vi "test_Create Data Channel_single channel type cast .vi"(8 "error in (no error)":errorcluster, 11 "TestCase in":refnum<class "Instrument Addon Scripting API Channels Unit Tests.lvclass">) -> (0 "error out":errorcluster, 3 "TestCase out":refnum<class "Instrument Addon Scripting API Channels Unit Tests.lvclass">)   [LabVIEW 2018, in "Instrument Addon Scripting API Channels Unit Tests.lvclass"]
uses:
  Instrument Addon Scripting API Channels Unit Tests.lvclass
  APIs/Scripting API/TypeDefs/Single Channel Type Cast Settings.ctl
  Addon/Addon Shared/Types/Type Cast Type.ctl
  Addon/Addon Shared/Types/Endian.ctl
  Addon/Addon Shared/Types/Protocol Data Type.ctl
  Addon/Addon Shared/Types/Data Channel Type.ctl
  Instrument Addon Scripting API Channels Unit Tests.lvclass/Instrument Addon Scripting API Channels Unit Tests.ctl
  Addon/Addon Shared/SubVIs/Constants.vi
  <vilib>/NI/NI VeriStand Advanced SysDef API/_SubVIs/SysDef.Search.GUID.vi
  <vilib>/NI/NI VeriStand Advanced SysDef API/_SubVIs/SysDef.Search.GUIDs.vi
  APIs/Scripting API/Channels/Create Data Channel - Single Channel - Type Cast.vi
  <vilib>/NI Veristand/Custom Device API/Get Item Property (U16).vi
  <vilib>/addons/_JKI Toolkits/VI Tester/TestCase.llb/TestCase.lvclass
  Instrument Addon Scripting API Test Assets/Instrument Addon Scripting API Test Assets.lvclass
  <vilib>/NI/NI VeriStand Advanced SysDef API/SysDef API/Advanced System Definition.lvlib
  Addon/Addon Shared/Instrument Addon Shared.lvlib
  <vilib>/NI Veristand/Custom Device API/Custom Device API.lvlib
  APIs/Scripting API/Instrument Addon Scripting API.lvlib
  C:/Program Files (x86)/National Instruments/LabVIEW 2018/vi.lib/addons/_JKI Toolkits/VI Tester/TestCase.llb/TestCase.lvclass
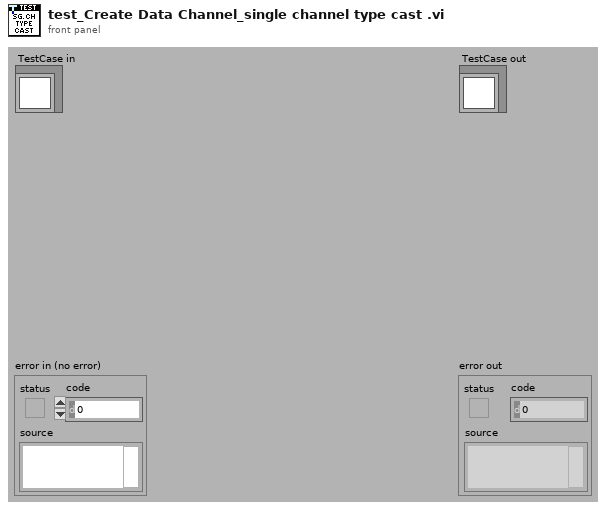
[diagram p1: front panel]
types:
  T1 = typedef "Instrument Addon Scripting API.lvlib/Single Channel Type Cast Settings.ctl" = cluster{"Type":T2, "Endian":T3, "Default Value":dbl, "Units":string}
  T2 = typedef "Instrument Addon Shared.lvlib/Type Cast Type.ctl" = enum16{"DBL", "SGL", "U64", "U32", "U16", "U8", "I64", "I32", "I16", "I8"}
  T3 = typedef "Instrument Addon Shared.lvlib/Endian.ctl" = enum16{"Native", "Little", "Big"}
  T4 = typedef "Instrument Addon Shared.lvlib/Data Channel Type.ctl" = enum16{"Format", "Comparison", "Type Cast", "Enumerated List"}
  T5 = typedef "Instrument Addon Shared.lvlib/Protocol Data Type.ctl" = enum16{"Single Channel", "Array"}
  T6 = typedef "Custom Device API.lvlib/Custom Device Item Ref.ctl" = u64
  T7 = typedef "Custom Device API.lvlib/Custom Device Channel.ctl" = cluster{"Type":T8, "Units":string, "Default Value":dbl, "Faultable":bool, "Scalable":bool}
  T8 = typedef "Custom Device API.lvlib/Custom Device Channel Type.ctl" = enum16{"Input", "Output"}
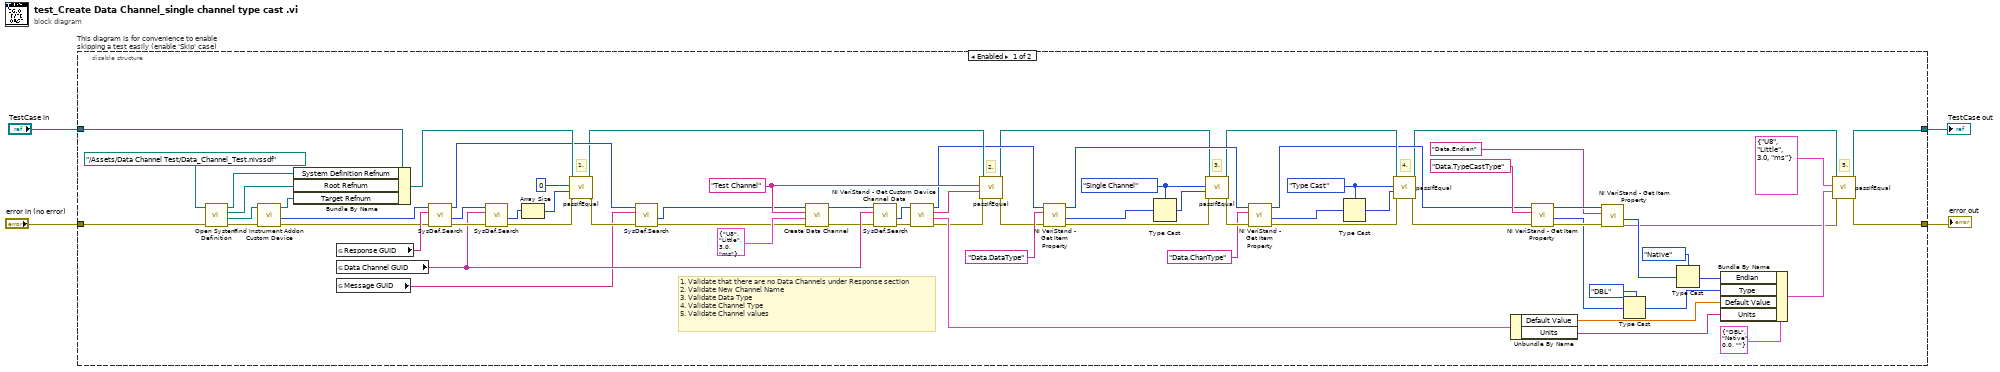
[diagram p0: block diagram]
diagram:
  n1 = disable-structure "This diagram is for convenience to enable skipping a test easily (enable 'Skip' case)" shown="Enabled" {
    disable-tunnel: "TestCase in" -> [w37 w79]
    disable-tunnel: [w75 w77] -> w1
    disable-tunnel: [w74 w78] -> w3
    disable-tunnel: "error in (no error)" -> [w70 w76]
    frame Enabled {
      w15 = Data_Channel_Type."Type Cast" ("Channel Type")
      w20 = Protocol_Data_Type."Single Channel" ("Data Type")
      w54 = "Test Channel" ("Name")
      # "2."
      # "4."
      # "3."
      # "5."
      # "1. Validate that there are no Data Channels under Response section\n2. Validate New Channel Name\n3. Validate Data Type\n4. Validate Channel Type\n5. Validate Channel values"
      # "1."
      n2 = call "Open System Definition.vi"("error in (no error)"=w70, "System Definition File"=path "../Assets/Data Channel Test/Data_Channel_Test.nivssdf") -> ("error out"=w73:errorcluster, "Target Refnum"=w72:refnum<k24>, "Root Refnum"=w34:refnum<k24>, "System Definition Refnum"=w36:refnum<k24>)  [unwired: 6 in]
      n3 = call "Find Instrument Addon Custom Device.vi"("error in"=w73, "target in"=w72) -> ("error out"=w38:errorcluster, "NodeID"=w30:u64, "target out"=w33:refnum<k24>)  [unwired: 7 in]
      n4 = Bundle By Name(cluster=w37, "System Definition Refnum"=w36, "Root Refnum"=w34, "Target Refnum"=w33) -> (w35:refnum<class "Instrument Addon Scripting API Channels Unit Tests.lvclass">)
      n5 = global read "Constants.vi" "Response GUID"() -> (w69:string)
      n6 = global read "Constants.vi" "Data Channel GUID"() -> (w66:string)
      n7 = global read "Constants.vi" "Message GUID"() -> (w31:string)
      n8 = call-poly <vilib>:"SysDef.Search.vi"("error in (no error)"=w38, "GUID"=w69, "nodeID"=w30) -> ("error out"=w67:errorcluster, "Value out"=w68:u64, "nodeID out"=w27:u64)  [unwired: 5 in, 1 out]
      n9 = call-poly <vilib>:"SysDef.Search.vi"("error in (no error)"=w67, "GUID"=w66, "nodeID"=w68) -> ("error out"=w58:errorcluster, "Values Out"=w57:u64[])  [unwired: 5 in, 2 out]
      n10 = Array Size(array=w57) -> (size(s)=w56:i32)
      n11 = call-dynamic "passIfEqual.vi"("error in (no error)"=w58, "y"=w56, "x"=0 ("size(s)"), "TestCase in"=w35) -> ("error out"=w32:errorcluster, "TestCase out"=w26:refnum<class "Instrument Addon Scripting API Channels Unit Tests.lvclass">)  [unwired: 6 in]
      n12 = call-poly <vilib>:"SysDef.Search.vi"("error in (no error)"=w32, "GUID"=w31, "nodeID"=w27) -> ("error out"=w29:errorcluster, "Value out"=w28:u64)  [unwired: 5 in, 2 out]
      n13 = call-poly "Create Data Channel.vi"("Error In"=w29, "Settings"=T1 {"Type"=enum."U8", "Endian"=enum."Little", "Default Value"=3.0, "Units"="ms"}, "Name"=w54, "Message Refnum In"=w28) -> ("Error Out"=w52:errorcluster, "Message Refnum Out"=w53:T6)  [unwired: 5 in, 1 out]
      n14 = call-poly <vilib>:"SysDef.Search.vi"("error in (no error)"=w52, "GUID"=w66, "nodeID"=w53) -> ("error out"=w65:errorcluster, "Value out"=w40:u64)  [unwired: 5 in, 2 out]
      n15 = call <vilib>:"NI VeriStand - Get Custom Device Channel Data.vi"("error in (no error)"=w65, "Channel Ref in"=w40) -> ("error out"=w25:errorcluster, "Channel"=w64:T7, "Channel Name"=w60:string, "Channel Ref out"=w12:T6)  [unwired: 4 in, 2 out]
      n16 = call-dynamic "passIfEqual.vi"("error in (no error)"=w25, "y"=w60, "x"=w54, "TestCase in"=w26) -> ("error out"=w11:errorcluster, "TestCase out"=w10:refnum<class "Instrument Addon Scripting API Channels Unit Tests.lvclass">)  [unwired: 6 in]
      n17 = call-poly <vilib>:"NI VeriStand - Get Item Property.vi"("error in (no error)"=w11, "Property Name"="Data.DataType", "Item Ref in"=w12) -> ("error out"=w23:errorcluster, "Value"=w22:u16, "Item Ref out"=w14:T6)  [unwired: 5 in, 1 out]
      n18 = Type Cast(type=w20, x=w22) -> (*(type *) &x=w21:T5)
      n19 = call-dynamic "passIfEqual.vi"("error in (no error)"=w23, "y"=w21, "x"=w20, "TestCase in"=w10) -> ("error out"=w19:errorcluster, "TestCase out"=w9:refnum<class "Instrument Addon Scripting API Channels Unit Tests.lvclass">)  [unwired: 6 in]
      n20 = call-poly <vilib>:"NI VeriStand - Get Item Property.vi"("error in (no error)"=w19, "Property Name"="Data.ChanType", "Item Ref in"=w14) -> ("error out"=w18:errorcluster, "Value"=w17:u16, "Item Ref out"=w8:T6)  [unwired: 5 in, 1 out]
      n21 = Type Cast(type=w15, x=w17) -> (*(type *) &x=w16:T4)
      n22 = call-dynamic "passIfEqual.vi"("error in (no error)"=w18, "y"=w16, "x"=w15, "TestCase in"=w9) -> ("error out"=w7:errorcluster, "TestCase out"=w6:refnum<class "Instrument Addon Scripting API Channels Unit Tests.lvclass">)  [unwired: 6 in]
      n23 = Unbundle By Name(w64) -> ("Default Value"=w63:dbl, "Units"=w62:string)
      n24 = call-poly <vilib>:"NI VeriStand - Get Item Property.vi"("error in (no error)"=w7, "Property Name"="Data.TypeCastType", "Item Ref in"=w8) -> ("error out"=w48:errorcluster, "Value"=w42:u16, "Item Ref out"=w49:T6)  [unwired: 5 in, 1 out]
      n25 = call-poly <vilib>:"NI VeriStand - Get Item Property.vi"("error in (no error)"=w48, "Property Name"="Data.Endian", "Item Ref in"=w49) -> ("error out"=w5:errorcluster, "Value"=w45:u16)  [unwired: 5 in, 2 out]
      n26 = Type Cast(type=Type_Cast_Type."DBL" ("Type"), x=w42) -> (*(type *) &x=w41:T2)
      n27 = Type Cast(type=Endian."Native" ("Endian"), x=w45) -> (*(type *) &x=w44:T3)
      n28 = Bundle By Name(cluster=T1 {"Type"=enum."DBL", "Endian"=enum."Native", "Default Value"=0.0, "Units"=""} ("Settings"), "Endian"=w44, "Type"=w41, "Default Value"=w63, "Units"=w62) -> (w59:T1)
      n29 = call-dynamic "passIfEqual.vi"("error in (no error)"=w5, "y"=w59, "x"=T1 {"Type"=enum."U8", "Endian"=enum."Little", "Default Value"=3.0, "Units"="ms"} ("Settings"), "TestCase in"=w6) -> ("error out"=w74:errorcluster, "TestCase out"=w75:refnum<class "Instrument Addon Scripting API Channels Unit Tests.lvclass">)  [unwired: 6 in]
    }
    frame Disabled {
      # "skip test result while test is under development"
      n30 = call <vilib>:"skip.vi"("error in (no error)"=w76, "TestCase in"=w79) -> ("error out"=w78:errorcluster, "TestCase out"=w77:refnum<class "Instrument Addon Scripting API Channels Unit Tests.lvclass">)  [unwired: 8 in]
    }
  }
  "error out" <- w3
  "TestCase out" <- w1
